vi "E Open.vi"(0 "File Path/表格路径":path, 1 "Visible/表格可见？(False)":bool, 5 "File Name/表格名称":string, 11 "Error In (no error)":errorcluster) -> (4 "Excel._Application":refnum<k7>, 6 "Excel._Workbook":refnum<k7>, 15 "Error Out":errorcluster)   [LabVIEW 2014]
doc: "打开指定路径下指定名称的电子表格，可以设置表格的可见或不可见。"
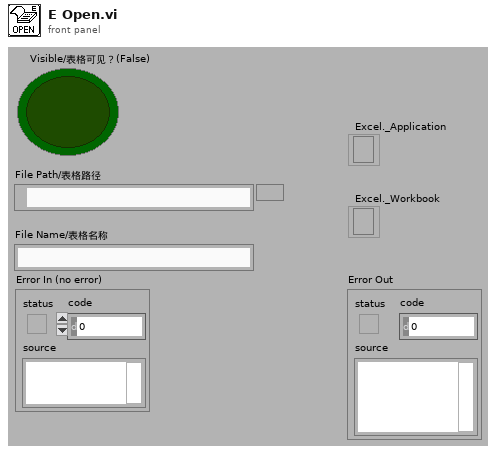
[diagram p1: front panel]
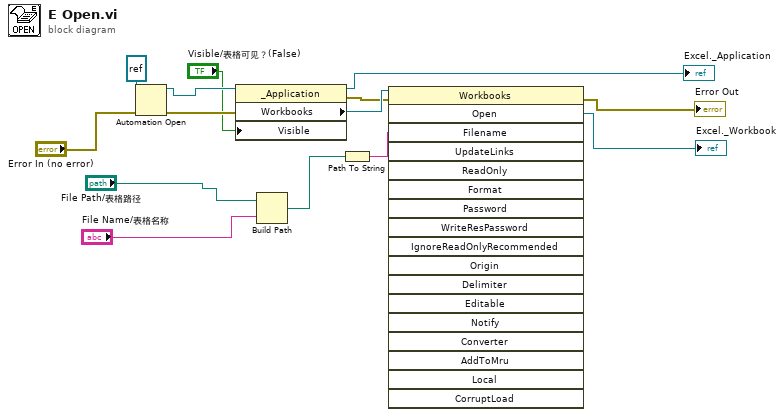
[diagram p0: block diagram]
diagram:
  n1 = Automation Open(error in (no error)="Error In (no error)", Automation Refnum=refnum<k7> refnum ("Excel._Application")) -> (Automation Refnum=w14:refnum<k7>, error out=w12:errorcluster)  [unwired: 2 in]
  n2 = property class="_Application"(reference=w14, error in=w12, "Visible"="Visible/表格可见？(False)") -> (reference out=→"Excel._Application":refnum<k7>, error out=w10:errorcluster, "Workbooks"=w13:refnum<k7>)
  n3 = Build Path(base path="File Path/表格路径", name or relative path="File Name/表格名称") -> (appended path=w9:path)
  n4 = Path To String(path=w9) -> (string=w8:string)
  n5 = invoke class="Workbooks" method="Open"(reference=w13, error in=w10, "Filename"=w8) -> (error out=→"Error Out":errorcluster, "Open"=→"Excel._Workbook":refnum<k7>)  [unwired: 15 in, 16 out]
